vi "orderbook.vi"(9 "Ready.For.OrderBook.Result":bool, 10 "OrderBook.Command.Valid":bool, 11 "OrderBook.Command":T1) -> (1 "Ready.for.OrderBook.Command":bool, 2 "OrderBook.Result.Valid":bool, 3 "OrderBook.Result":T3)   [LabVIEW 2020]
uses:
  application/orderbook.result.type.ctl
  application/orderbook.result.ctl
  orderbook.state.ctl
  orderbook.command.type.ctl
  orderbook.command.ctl
panel:
  in  "Reset":bool
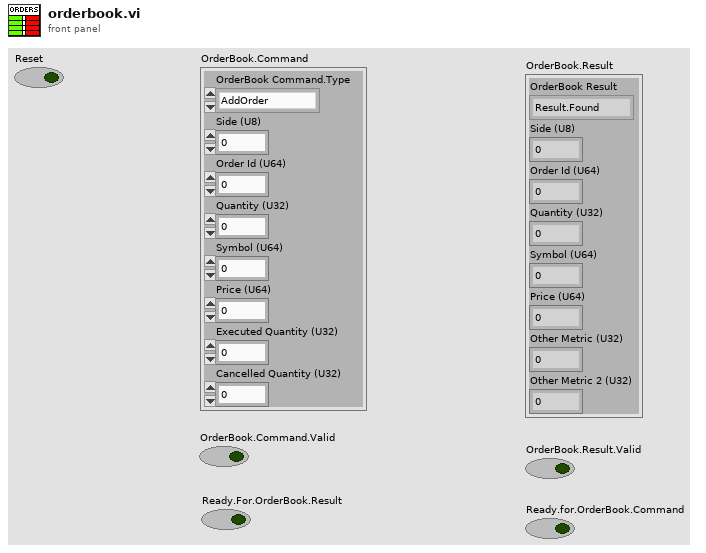
[diagram p1: front panel]
types:
  T1 = typedef "orderbook.command.ctl" = cluster{"OrderBook Command.Type":T2, "Side (U8)":u8, "Order Id (U64)":u64, "Quantity (U32)":u32, "Symbol (U64)":u64, "Price (U64)":u64, "Executed Quantity (U32)":u32, "Cancelled Quantity (U32)":u32}
  T2 = typedef "orderbook.command.type.ctl" = enum16{"AddOrder", "OrderExecuted", "ReduceSize", "ModifyOrder", "DeleteOrder", "Query"}
  T3 = typedef "orderbook.result.ctl" = cluster{"OrderBook Result":T4, "Side (U8)":u8, "Order Id (U64)":u64, "Quantity (U32)":u32, "Symbol (U64)":u64, "Price (U64)":u64, "Other Metric (U32)":u32, "Other Metric 2 (U32)":u32}
  T4 = typedef "orderbook.result.type.ctl" = enum16{"Result.Found", "Result.Not.Found"}
  T5 = typedef "orderbook.state.ctl" = enum16{"Reset", "WaitForNewCommand", "AddOrder", "Query"}
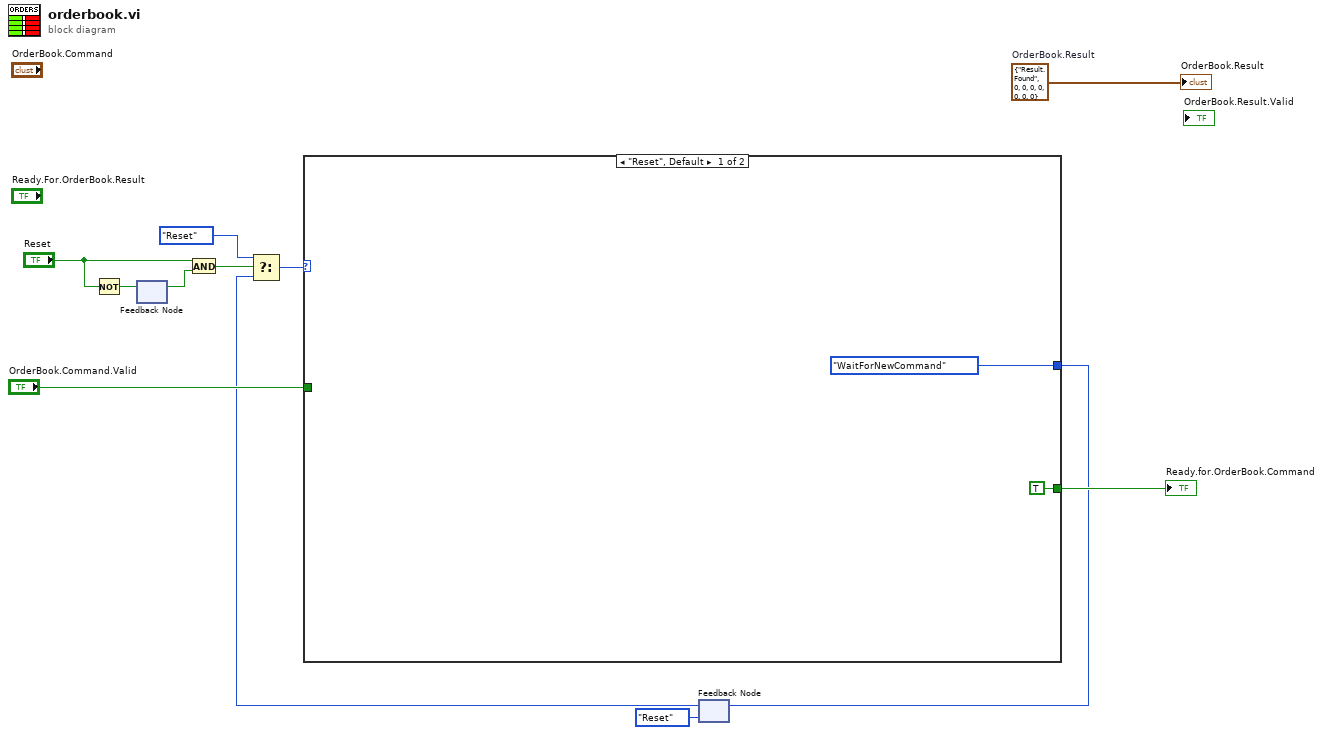
[diagram p0: block diagram]
diagram:
  w12 = T3 {"OrderBook Result"=enum."Result.Found", "Side (U8)"=0, "Order Id (U64)"=0, "Quantity (U32)"=0, "Symbol (U64)"=0, "Price (U64)"=0, "Other Metric (U32)"=0, "Other Metric 2 (U32)"=0}  # OrderBook.Result
  n1 = Not(x="Reset") -> (.not. x?=w7:bool)
  n2 = feedback-in #1(w7) -> ()
  n3 = feedback #1() -> (w8:bool)  [unwired: 1 in]
  n4 = And(x="Reset", y=w8) -> (x .and. y?=w5:bool)
  n5 = feedback #2(orderbook.state."Reset" ("OrderBook.State")) -> (w4:T5)
  n6 = Select(t=orderbook.state."Reset" ("OrderBook.State"), s=w5, f=w4) -> (s? t:f=w3:T5)
  n7 = case shown="\"Reset\", Default" w3 {
    tunnel: "OrderBook.Command.Valid" -> [_ _]
    tunnel: [TRUE _] -> w10
    tunnel: [orderbook.state."WaitForNewCommand" ("OrderBook.State") _] -> w9
    frame "Reset", Default {
    }
    frame "AddOrder" {
    }
  }
  "Ready.for.OrderBook.Command" <- w10
  n8 = feedback-in #2(w9) -> ()
  "OrderBook.Result" <- w12
